vi "Scroll Message to String Array.vi"(7 "Scroll Text":string) -> (8 "Array":string[](array[string]))   [LabVIEW 2016, in "TLMB.lvlib"]
uses:
  Projects/TLMB.lvlib
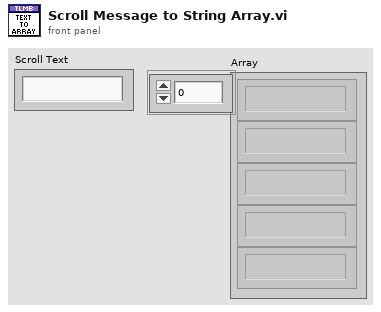
[diagram p1: front panel]
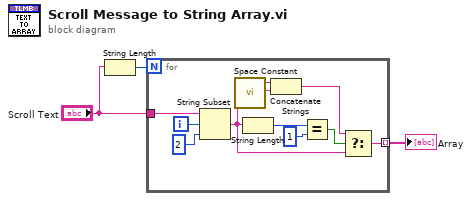
[diagram p0: block diagram]
diagram:
  n1 = String Length(string="Scroll Text") -> (length=w1:i32)
  n2 = for {
    N: w1 -> [_]
    tunnel: "Scroll Text" -> [w13]
    tunnel: [w7] -> w3 mode=indexing
    i -> [w11]
    n3 = String Subset(string=w13, offset (0)=w11, length (rest)=2 ("length (rest)")) -> (substring=w6:string)
    n4 = call <vilib>:"Space Constant.vi"() -> ("String"=w5:string)
    n5 = String Length(string=w6) -> (length=w10:i32)
    n6 = Concatenate Strings(w6, w5) -> (w4:string)
    n7 = Equal?(x=w10, y=1) -> (x = y?=w8:bool)
    n8 = Select(t=w4, s=w8, f=w6) -> (s? t:f=w7:string)
  }
  "Array" <- w3
